vi "滤波 (子VI).vi"(5 "滤波器选择":u16(ring) items=["切比雪夫", "巴特沃斯", "无"], 6 "阶数":dbl=2.0 format="%.2f", 7 "滤波器类型":i32(ring) items=["低通", "高通", "带通", "带阻"], 8 "采样率":u32=8000, 9 "低截止频率":dbl=60.0 format="%.2f", 10 "高截止频率":dbl=8000.0 format="%.2f", 11 "X输入":dbl[](array[numeric])) -> (3 "滤波输出":dbl[](array[numeric]))   [LabVIEW 2014]
uses:
  <vilib>/Analysis/3filter.llb/Chebyshev Filter (DBL).vi
  <vilib>/Analysis/3filter.llb/Butterworth Filter (DBL).vi
  <vilib>/Analysis/NI_AALBase.lvlib
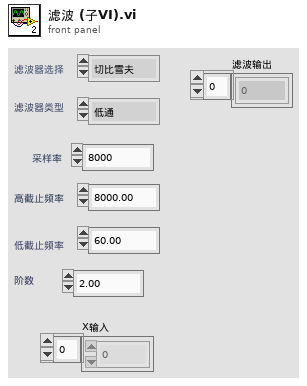
[diagram p1: front panel]
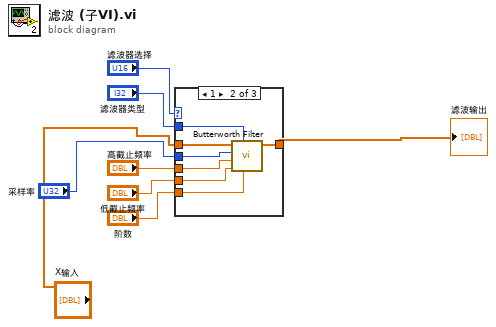
[diagram p0: block diagram]
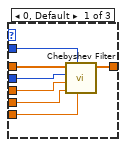
[diagram p2: hidden frame]
diagram:
  n1 = case shown="1" "滤波器选择" {
    tunnel: "滤波器类型" -> [w10 w22 _]
    tunnel: "高截止频率" -> [w15 w19 _]
    tunnel: "低截止频率" -> [w14 w18 _]
    tunnel: "阶数" -> [w13 w17 _]
    tunnel: "采样率" -> [w12 w20 _]
    tunnel: "X输入" -> [w11 w21 w23]
    tunnel: [w9 w16 w23] -> w8
    frame 0, Default {
      n2 = call-poly <vilib>:"Chebyshev Filter.vi"("ripple(dB)"=w13, "filter type"=w10, "low cutoff freq: fl"=w14, "high cutoff freq: fh"=w15, "sampling freq: fs"=w12, "X"=w11) -> ("Filtered X"=w9:dbl[])  [unwired: 4 in, 1 out]
    }
    frame 1 {
      n3 = call-poly <vilib>:"Butterworth Filter.vi"("order"=w17, "filter type"=w22, "low cutoff freq: fl"=w18, "high cutoff freq: fh"=w19, "sampling freq: fs"=w20, "X"=w21) -> ("Filtered X"=w16:dbl[])  [unwired: 2 in, 1 out]
    }
    frame 2 {
    }
  }
  "滤波输出" <- w8
